vi "Render Inverted Section with Empty Array Object.vi"(8 "Error In":errorcluster) -> (0 "Error Out":errorcluster)   [LabVIEW 2018, in "Tests.lvlib" / "Render.lvlib"]
uses:
  Render.lvlib
  <vilib>/addons/_JKI Toolkits/Caraya/classes/Test/Test.lvclass
  <vilib>/addons/_JKI Toolkits/Caraya/classes/Assert/Assert.lvclass
  src/Toolkit/Toolkit.lvlib
  src/Toolkit/Data/Map/Map.lvclass
  src/Toolkit/Low-Level/Support/Lex String.vi
  src/Toolkit/Data/Map/Support/From Datum.vi
  src/Toolkit/Low-Level/Support/Render to String.vi
  src/Toolkit/Data/Array/Array.lvclass
  src/Toolkit/Data/Array/Support/From Strings.vi
  src/Toolkit/Low-Level/Context/Compiler.lvclass
  D:/Users/cfield/Code/Field R&D Services/Labstache/src/Toolkit/Data/Datum/Datum.lvclass
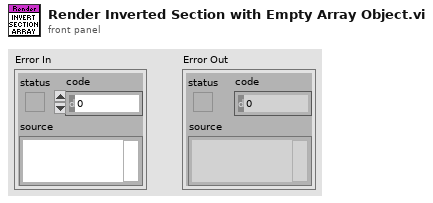
[diagram p1: front panel]
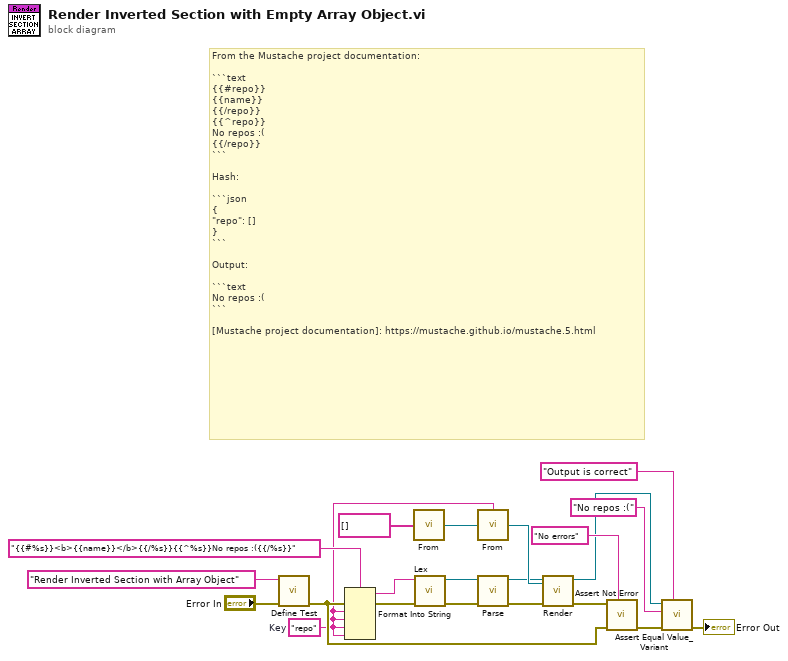
[diagram p0: block diagram]
diagram:
  w4 = "repo"  # Key
  # "From the Mustache project documentation:\n\n```text\n{{#repo}}\n{{name}}\n{{/repo}}\n{{^repo}}\nNo repos :(\n{{/repo}}\n```\n\nHash:\n\n```json\n{\n\"repo\": []\n}\n```\n\nOutput:\n\n```text\nNo repos :(\n```\n\n[Mustache project documentation]: https://mustache.github.io/mustache.5.html"
  n1 = call <vilib>:"Define Test.vi"("error in (no error)"="Error In", "Label (VI Title)"="Render Inverted Section with Array Object") -> ("error out"=w9:errorcluster)  [unwired: 9 in]
  n2 = Format Into String(format string="{{#%s}}<b>{{name}}</b>{{/%s}}{{^%s}}No repos :({{/%s}}", error in=w9, w4, w4, w4, w4) -> (resulting string=w6:string, error out=w8:errorcluster)  [unwired: 1 in]
  n3 = call-poly "From.vi"("Strings"=string[] []) -> ("Array"=w2:refnum<class "Array.lvclass">)  [unwired: 1 in]
  n4 = call-poly "Lex.vi"("Error In"=w8, "Context In"=w6) -> ("Error Out"=w11:errorcluster, "Context Out"=w12:refnum<class "Compiler.lvclass">)  [unwired: 7 in, 1 out]
  n5 = call-poly "From.vi"("Value"=w2, "Key"=w4) -> ("Map"=w10:refnum<class "Map.lvclass">)
  n6 = call "Parse.vi"("Error In"=w11, "Context In"=w12) -> ("Error Out"=w13:errorcluster, "Context Out"=w3:refnum<class "Compiler.lvclass">)  [unwired: 7 in, 1 out]
  n7 = call-poly "Render.vi"(7:w10, "Error In"=w13, "Context In"=w3) -> ("Error Out"=w15:errorcluster, "Context Out"=w14:refnum<class "Compiler.lvclass">)  [unwired: 6 in, 1 out]
  n8 = call <vilib>:"Assert Not Error.vi"("Label"="No errors", "error in (no error)"=w9, "Not Error?"=w15) -> ("error out"=w18:errorcluster)  [unwired: 8 in]
  n9 = call <vilib>:"Assert Equal Value_Variant.vi"("Label"="Output is correct", "error in (no error)"=w18, "Y"="No repos :(", "X"=w14) -> ("error out"=→"Error Out":errorcluster)  [unwired: 7 in]
